vi "ActionVIOnCompile.vi"(8 "error in (no error)":errorcluster, 11 "Device Item Ref in":T1 format="%.0x") -> (0 "error out":errorcluster)   [LabVIEW 2018, in "Vires VTD System Explorer.lvlib"]
uses:
  Vires VTD System Explorer.lvlib
  <vilib>/NI Veristand/Custom Device API/Custom Device Item Ref.ctl
  Shared/Compiled.Settings.ctl
  RDB Data.ctl
  RDB/RDB Object.ctl
  RDB/RDB Player Object.ctl
  Shared/Network Settings.ctl
  Shared/Protocol.ctl
  Shared/SensorInfos.ctl
  Shared/SensorInfo.ctl
  Shared/Sensor Name.ctl
  MM/MM Data.ctl
  MM/MM Objects.ctl
  MM/MM Object.ctl
  Shared/Constants.vi
  <vilib>/NI Veristand/Custom Device Tools/Custom Device Utility Library/NI VeriStand - Search for Item by Name.vi
  <vilib>/NI Veristand/Custom Device API/Get Item Property (Variant).vi
  <vilib>/NI Veristand/Custom Device API/Set Item Property (Variant).vi
  <vilib>/NI Veristand/Custom Device API/Custom Device API.lvlib
  <vilib>/NI Veristand/Custom Device Tools/Custom Device Utility Library/Custom Device Utility Library.lvlib
  <vilib>/NI/NIVS Inline Async API/_Data Access System Explorer/Data Access System Explorer.lvlib
  Shared/Vires VTD Shared.lvlib
  RDB/RDB.lvlib
  MM/MM.lvlib
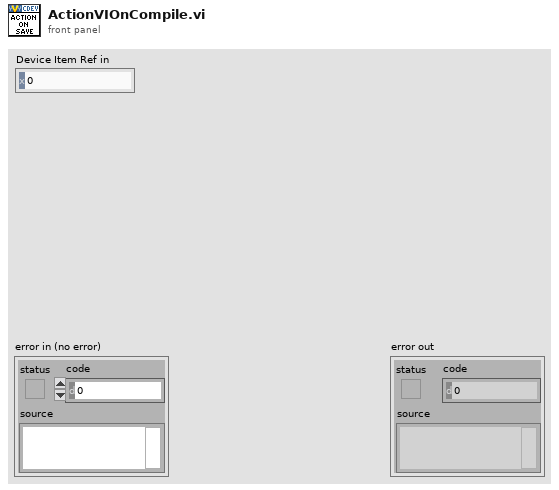
[diagram p1: front panel]
types:
  T1 = typedef "Custom Device API.lvlib/Custom Device Item Ref.ctl" = u64
  T2 = cluster{"Name":string, "Type":enum16{"Output/Write", "Input/Read", "Input/ReadWrite"}, "VS Refs":T1[]}
  T3 = enum16{"Output/Write", "Input/Read", "Input/ReadWrite"}
  T4 = typedef "Vires VTD Shared.lvlib/Compiled.Settings.ctl" = cluster{"Name":string, "RDB Data Receive ":T5, "RDB Data Sent":T5, "vclient":path, "Network Settings":T8, "SensorInfos":T10, "mmanager":path, "Scenario Paths":string[], "Custom SCP Commands":string[]}
  T5 = typedef "Vires VTD Shared.lvlib/RDB Data.ctl" = T6[]
  T6 = typedef "RDB.lvlib/RDB Object.ctl" = cluster{"pkID":i32, "RDB Player Objects":T7[]}
  T7 = typedef "RDB.lvlib/RDB Player Object.ctl" = cluster{"PlayerID":i32, "Signals":string[], "WheelID":i32}
  T8 = typedef "Vires VTD Shared.lvlib/Network Settings.ctl" = cluster{"IP adress":string, "RDB":cluster{"Protocol":T9, "Tx Port":u16, "Rx Port":u16, "Buffer Size":i32, "Timeout":u16}, "SCP":cluster{"Protocol":T9, "Tx Port":u16, "Rx Port":u16, "Buffer Size":i32, "Timeout":u16}}
  T9 = typedef "Vires VTD Shared.lvlib/Protocol.ctl" = enum16{"UDP", "TCP"}
  T10 = typedef "Vires VTD Shared.lvlib/SensorInfos.ctl" = T11[]
  T11 = typedef "Vires VTD Shared.lvlib/SensorInfo.ctl" = cluster{"Sensor Name":T12, "Protocol":T9, "Network port":i32, "# Culled Objects":i32, "PlayerID":u8, "MM Data":T13}
  T12 = typedef "Vires VTD Shared.lvlib/Sensor Name.ctl" = string
  T13 = typedef "Vires VTD Shared.lvlib/MM Data.ctl" = T14[]
  T14 = typedef "MM.lvlib/MM Objects.ctl" = cluster{"pkID":i32, "MM Objects":T15[]}
  T15 = typedef "MM.lvlib/MM Object.ctl" = cluster{"Object":i32, "Signals":string[]}
  T16 = typedef "Custom Device API.lvlib/Custom Device Item Info.ctl" = cluster{"Name":string, "Is Channel":bool, "GUID":string, "Is Waveform":bool}
  T17 = cluster{"Name":string, "Type":enum16{"Output/Write", "Input/Read", "Input/ReadWrite"}, "VS Refs":T1[]}[]
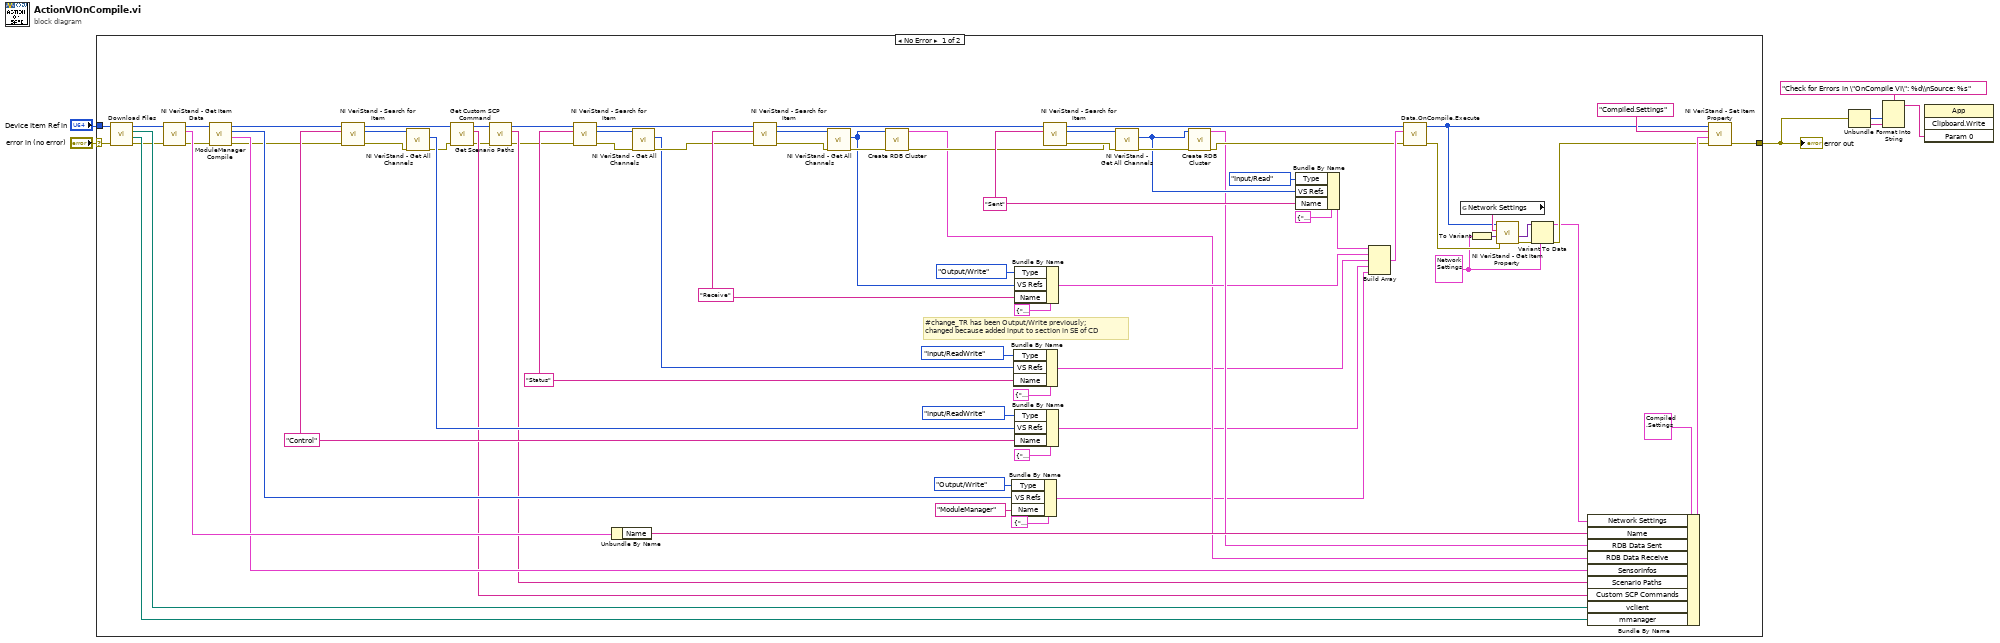
[diagram p0: block diagram]
diagram:
  n1 = case shown="No Error" "error in (no error)" {
    selector: "error in (no error)" -> [w55 w86]
    tunnel: [w57 w86] -> w3
    tunnel: "Device Item Ref in" -> [w56 _]
    frame No Error {
      w20 = "Control" ("Item Name")
      w42 = "Status" ("Item Name")
      w31 = T8 {"IP adress"="127.0.0.1", "RDB"={"Protocol"=enum."UDP", "Tx Port"=48190, "Rx Port"=8192, "Buffer Size"=48190, "Timeout"=10}, "SCP"={"Protocol"=enum."UDP", "Tx Port"=48190, "Rx Port"=8192, "Buffer Size"=48190, "Timeout"=10}} ("UDP Settings")
      w80 = "Sent" ("Item Name")
      w81 = "Receive" ("Item Name")
      # "#change_TR has been Output/Write previously;\nchanged because added input to section in SE of CD"
      n2 = call "Download Files.vi"("error in (no error)"=w55, "Item Ref in"=w56) -> ("error out"=w10:errorcluster, "mmanager"=w32:path, "vclient"=w34:path, "Device Ref out"=w54:T1)  [unwired: 6 in]
      n3 = call <vilib>:"NI VeriStand - Get Item Data.vi"("error in (no error)"=w10, "Item Ref in"=w54) -> ("error out"=w39:errorcluster, "Item Info"=w83:T16, "Item Ref out"=w40:T1)  [unwired: 6 in, 1 out]
      n4 = call "ModuleManager Compile.vi"("error in"=w39, "Section Ref in"=w40) -> ("error out"=w18:errorcluster, "SensorInfos"=w33:T10, "Channel Refs"=w36:T1[], "Section Ref out"=w21:T1)  [unwired: 6 in]
      n5 = call-poly <vilib>:"NI VeriStand - Search for Item.vi"("error in"=w18, "Item Name"=w20, "Section Ref in"=w21) -> ("error out"=w23:errorcluster, "Item Ref"=w22:T1, "Section Ref out"=w14:T1)  [unwired: 5 in, 1 out]
      n6 = call <vilib>:"NI VeriStand - Get All Channels.vi"("error in"=w23, "Section Ref in"=w22) -> ("error out"=w17:errorcluster, "Channel Refs"=w19:T1[])  [unwired: 6 in, 2 out]
      n7 = call "Get Custom SCP Command.vi"("error in (no error)"=w17, "Section Ref in"=w14) -> ("error out"=w8:errorcluster, "Custom SCP Commands (str)"=w12:string[], "Section Ref out"=w13:T1)  [unwired: 7 in]
      n8 = call "Get Scenario Paths.vi"("error in (no error)"=w8, "Section Ref in"=w13) -> ("error out"=w9:errorcluster, "Scenario Paths (str)"=w11:string[], "Section Ref out"=w16:T1)  [unwired: 6 in, 1 out]
      n9 = call-poly <vilib>:"NI VeriStand - Search for Item.vi"("error in"=w9, "Item Name"=w42, "Section Ref in"=w16) -> ("error out"=w48:errorcluster, "Item Ref"=w49:T1, "Section Ref out"=w47:T1)  [unwired: 5 in, 1 out]
      n10 = Unbundle By Name(w83) -> ("Name"=w82:string)
      n11 = call <vilib>:"NI VeriStand - Get All Channels.vi"("error in"=w48, "Section Ref in"=w49) -> ("error out"=w46:errorcluster, "Channel Refs"=w43:T1[])  [unwired: 6 in, 2 out]
      n12 = call-poly <vilib>:"NI VeriStand - Search for Item.vi"("error in"=w46, "Item Name"=w81, "Section Ref in"=w47) -> ("error out"=w70:errorcluster, "Item Ref"=w69:T1, "Section Ref out"=w72:T1)  [unwired: 5 in, 1 out]
      n13 = call <vilib>:"NI VeriStand - Get All Channels.vi"("error in"=w70, "Section Ref in"=w69) -> ("error out"=w66:errorcluster, "Channel Refs"=w65:T1[])  [unwired: 6 in, 2 out]
      n14 = call "Create RDB Cluster.vi"("error out"=w66, "Channel Refs"=w65) -> ("error out 2"=w64:errorcluster, "Array"=w58:T5)  [unwired: 8 in]
      n15 = Bundle By Name(cluster=T2 {"Name"="", "Type"=enum."Output/Write", "VS Refs"=[]} ("Group"), "Type"=T3."Output/Write", "VS Refs"=w36, "Name"="ModuleManager") -> (w27:T2)
      n16 = Bundle By Name(cluster=T2 {"Name"="", "Type"=enum."Output/Write", "VS Refs"=[]} ("Group"), "Type"=T3."Input/ReadWrite", "VS Refs"=w43, "Name"=w42) -> (w41:T2)
      n17 = Bundle By Name(cluster=T2 {"Name"="", "Type"=enum."Output/Write", "VS Refs"=[]} ("Group"), "Type"=T3."Output/Write", "VS Refs"=w65, "Name"=w81) -> (w59:T2)
      n18 = Bundle By Name(cluster=T2 {"Name"="", "Type"=enum."Output/Write", "VS Refs"=[]} ("Group"), "Type"=T3."Input/ReadWrite", "VS Refs"=w19, "Name"=w20) -> (w24:T2)
      n19 = call-poly <vilib>:"NI VeriStand - Search for Item.vi"("error in"=w64, "Item Name"=w80, "Section Ref in"=w72) -> ("error out"=w68:errorcluster, "Item Ref"=w67:T1, "Section Ref out"=w73:T1)  [unwired: 5 in, 1 out]
      n20 = call <vilib>:"NI VeriStand - Get All Channels.vi"("error in"=w68, "Section Ref in"=w67) -> ("error out"=w63:errorcluster, "Channel Refs"=w62:T1[])  [unwired: 6 in, 2 out]
      n21 = call "Create RDB Cluster.vi"("error out"=w63, "Channel Refs"=w62) -> ("error out 2"=w61:errorcluster, "Array"=w60:T5)  [unwired: 8 in]
      n22 = Bundle By Name(cluster=T2 {"Name"="", "Type"=enum."Output/Write", "VS Refs"=[]} ("Group"), "Type"=T3."Input/Read", "VS Refs"=w62, "Name"=w80) -> (w78:T2)
      n23 = Build Array(w78, w59, w41, w24, w27) -> (w76:T17)
      n24 = call <vilib>:"Data.OnCompile.Execute.vi"("error in"=w61, "VS Ref Groups"=w76, "Custom Device Ref"=w73) -> ("error out"=w50:errorcluster, "Custom Device Ref"=w29:T1)  [unwired: 7 in]
      n25 = global read "Constants.vi" "Network Settings"() -> (w53:string)
      n26 = To Variant(anything=w31) -> (Variant=w30:variant)
      n27 = call-poly <vilib>:"NI VeriStand - Get Item Property.vi"("error in (no error)"=w50, "Default Value"=w30, "Property Name"=w53, "Item Ref in"=w29) -> ("error out"=w52:errorcluster, "Value"=w51:variant)  [unwired: 4 in, 2 out]
      n28 = Variant To Data(error in=w52, type=w31, Variant=w51) -> (data=w15:T8, error out=w28:errorcluster)
      n29 = Bundle By Name(cluster=T4 {"Name"="", "RDB Data Receive "=[], "RDB Data Sent"=[], "vclient"=path "", "Network Settings"={"IP adress"="127.0.0.1", "RDB"={"Protocol"=enum."UDP", "Tx Port"=48190, "Rx Port"=10, "Buffer Size"=204800, "Timeout"=10}, "SCP"={"Protocol"=enum."TCP", "Tx Port"=48191, "Rx Port"=48191, "Buffer Size"=204800, "Timeout"=10}}, "SensorInfos"=[], "mmanager"=path "", "Scenario Paths"=[], "Custom SCP Commands"=[]} ("Compiled.Settings"), "Network Settings"=w15, "Name"=w82, "RDB Data Sent"=w60, "RDB Data Receive"=w58, "SensorInfos"=w33, "Scenario Paths"=w11, "Custom SCP Commands"=w12, "vclient"=w34, "mmanager"=w32) -> (w84:T4)
      n30 = call-poly <vilib>:"NI VeriStand - Set Item Property.vi"("error in (no error)"=w28, "Value"=w84, "Property Name"="Compiled.Settings", "Item Ref in"=w29) -> ("error out"=w57:errorcluster)  [unwired: 5 in, 2 out]
    }
    frame Error {
    }
  }
  "error out" <- w3
  n31 = Unbundle(w3) -> ("code"=w4:i32, "source"=w5:string)  [unwired: 1 out]
  n32 = Format Into String(format string="Check for Errors in \"OnCompile VI\": %d\\nSource: %s", w4, w5) -> (resulting string=w2:string)  [unwired: 2 in, 1 out]
  n33 = invoke class="App" method="Clipboard.Write"("Param 0"=w2) -> ()  [unwired: 3 in, 4 out]
